vi "GV_Constructor.vi"(4 "Graph-ref":refnum<vi>, 5 "menu reference":refnum<k9>, 6 "StartupTagList":string[](array[string]), 7 "Pane":refnum<vi>, 8 "error in (no error)":errorcluster, 9 "Gserver-Queue":refnum<queue>, 10 "GviewName":string, 11 "Gviewer in":refnum<class "Gviewer.lvclass">) -> (0 "error out":errorcluster, 3 "Gviewer out":refnum<class "Gviewer.lvclass">)   [LabVIEW 2020, in "Sgraph_lib_V1.lvlib" / "Gviewer.lvclass"]
doc: "Constructor of the Sgraph Viewer : Set all default values, connect to Vserver, Setup default start conditions"
uses:
  Gviewer.lvclass
  Gserver/controls/Typedef_Gviewer-Query.ctl
  Gserver/controls/Typedef_QueryType.ctl
  Gviewer.lvclass/Gviewer.ctl
  <vilib>/Utility/miscctls.llb/LVPointTypeDef.ctl
  controls/ToolBarAppearance.ctl
  <vilib>/Utility/miscctls.llb/LVPositionTypeDef.ctl
  controls/Typedef_Gserver-Replies.ctl
  controls/Typedef_ServerActions.ctl
  FAMM/controls/Typedef_Gviewer_TagsUnits.ctl
  Common/controls/typedef_com_TagProp.ctl
  controls/TD_Lscale.ctl
  controls/TD_Rscale.ctl
  controls/Typedef_Live.ctl
  controls/MinMax.ctl
  controls/Typedef_ZoomEvent.ctl
  controls/Typedef_SelProperties.ctl
  controls/Typedef_LineType.ctl
  Gserver/Gserver.lvclass
  Builds/Sgraph_lib_V1.lvlib
  FAMM/FAMM.lvclass
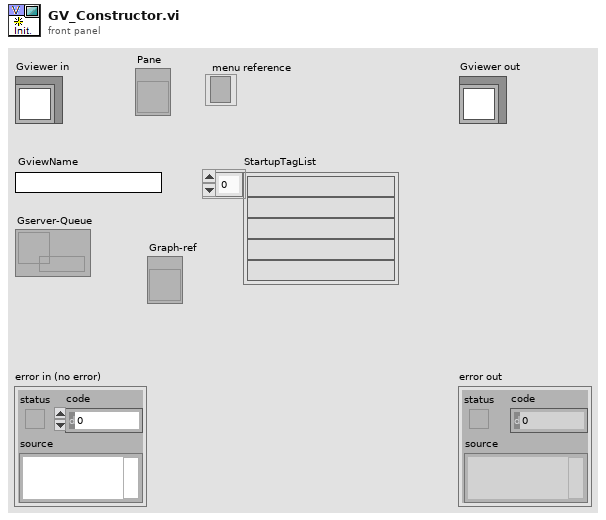
[diagram p1: front panel]
types:
  T1 = typedef "Sgraph_lib_V1.lvlib/Gviewer.lvclass/ToolBarAppearance.ctl" = enum16{"Bare", "Native", "Gradient"}
  T2 = typedef "LVPointTypeDef.ctl" = cluster{"Horizontal":i16, "Vertical":i16}
  T3 = typedef "LVPositionTypeDef.ctl" = cluster{"Left":i32, "Top":i32}
  T4 = typedef "Typedef_Gserver-Replies.ctl" = cluster{"ServerActions":T5, "data":variant, "Source":string, "Time Stamp":timestamp}
  T5 = typedef "Sgraph_lib_V1.lvlib/Gviewer.lvclass/Typedef_ServerActions.ctl" = enum16{"GraphUpdate", "SendAllTags", "SendIniPath", "SetGeneralOptions", "EditTagsOpen", "EditTagsPresetSave", "EditTagsPresetLoad", "EditTagsClose", "NewTagSelection", "AutoScale", "DBeditStatus", "DBsaveConfirm", "ExitGraph"}
  T6 = typedef "Sgraph_lib_V1.lvlib/Gserver.lvclass/Typedef_QueryType.ctl" = enum16{"Subscribe", "DataRequest", "RequestAllTags", "RequestIniPath", "FAMMstarted", "SetClientOptions", "GviewerUpdate", "OpenNewGraph", "CloseClient", "CloseAllClients", "Close Gserver", "OpenMemoryMap", "MeMapDataRequest", "MeMapDataResponse", "OpenDBeditor", "CheckDBeditorRunning", "StoppedDBeditor", "SaveDB_TAGpropRecord", "ConfirmDB_TAGpropSave"}
  T7 = typedef "Sgraph_lib_V1.lvlib/Gserver.lvclass/Typedef_Gviewer-Query.ctl" = cluster{"Query_type":T6, "data":variant, "Source":string, "Time Stamp":timestamp}
  T8 = enum32{"Invalid", "Standard", "Closed", "Hidden", "Minimized", "Maximized"}
  T9 = typedef "Sgraph_lib_V1.lvlib/FAMM.lvclass/Typedef_Gviewer_TagsUnits.ctl" = cluster{"PAQ_TAGs":string[], "WAQ_TAGs":string[], "EAQ_TAGs":string[], "PAQtagProps":T10[], "WAQtagProps":T10[], "EAQtagProps":T10[]}
  T10 = typedef "Sgraph_lib_V1.lvlib/typedef_com_TagProp.ctl" = cluster{"Description":string, "EngUnits":string, "RangeH":dbl, "RangeL":dbl, "Resolution":i32, "Obsolete":bool, "ChangeDate":timestamp, "ChangeSource":string, "ChangeReason":string, "TagFunc":u32}
  T11 = typedef "Sgraph_lib_V1.lvlib/Gviewer.lvclass/TD_Rscale.ctl" = enum16{"none", "one", "all"}
  T12 = typedef "Sgraph_lib_V1.lvlib/Gviewer.lvclass/TD_Lscale.ctl" = enum16{"none", "one", "many"}
  T13 = typedef "Sgraph_lib_V1.lvlib/Gviewer.lvclass/Typedef_Live.ctl" = enum16{"Live View", "Freeze"}
  T14 = typedef "Sgraph_lib_V1.lvlib/Gviewer.lvclass/MinMax.ctl" = enum16{"On", "Off", "Focus"}
  T15 = typedef "MenuStructure.ctl" = cluster{"After_tag":string, "MenuItems":T16[]}[]
  T16 = typedef "MenuItem.ctl" = cluster{"name":string, "tag":string, "checked":bool, "enabled":bool}
  T17 = typedef "Sgraph_lib_V1.lvlib/Gviewer.lvclass/Typedef_ZoomEvent.ctl" = cluster{"Time-Start":timestamp, "Time-End":timestamp, "TimeSpan(sec)":dbl, "Live":T13, "SelProperties":T18[], "Time Stamp":timestamp}
  T18 = typedef "Sgraph_lib_V1.lvlib/Gviewer.lvclass/Typedef_SelProperties.ctl" = cluster{"Color":u32, "LineType":T19, "max":dbl, "min":dbl, "unit":string}
  T19 = typedef "Sgraph_lib_V1.lvlib/Gviewer.lvclass/Typedef_LineType.ctl" = enum16{"num_bare", "num_MinMax_Area", "num_MinMax_Lines", "num_MinMax_Forfor", "num_Max_Area", "num_Max_Line", "num_Max_Forfor", "num_Min_Area", "num_Min_Line", "num_Min_Fosfor", "Boolean_Line_01", "Boolean_Area_01", "Boolean_Fosfor_01", "Boolean_Line_TF", "Boolean_Area_TF", "Boolean_Fosfor_TF", "Boolean_OnOff_Line", "Boolean_OnOff_Area", "Boolean_OnOff_Fosfor", "Boolean_spare", "StringEvent_Line", "StringEvent_TimeLine"}
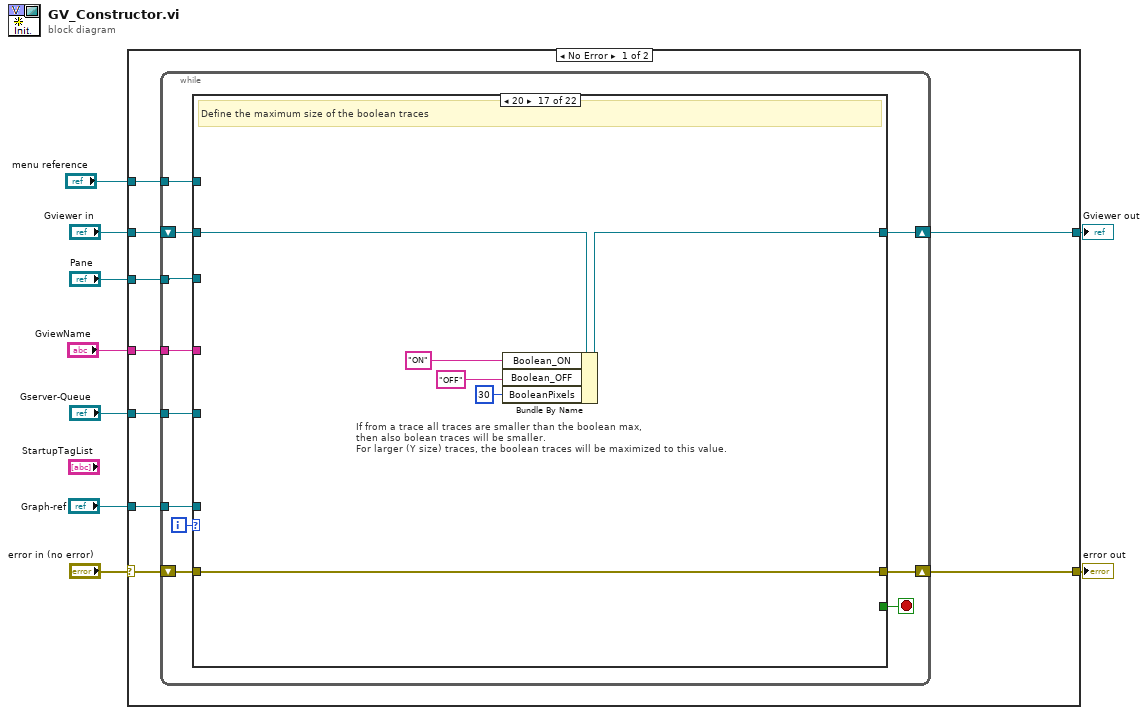
[diagram p0: block diagram]
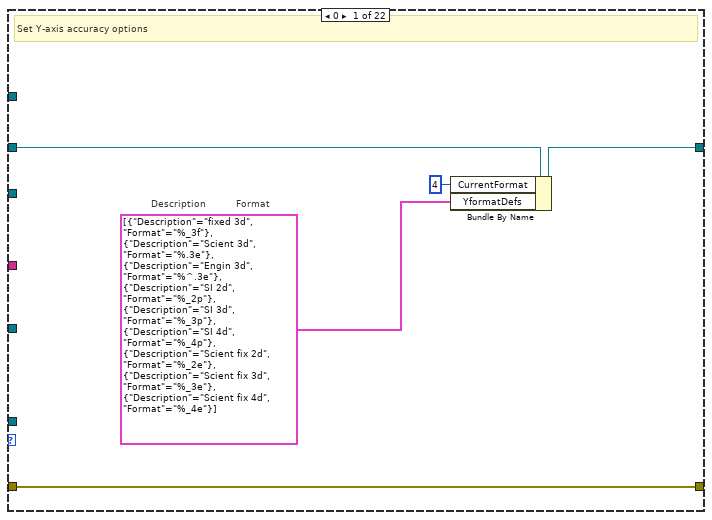
[diagram p2: hidden frame]
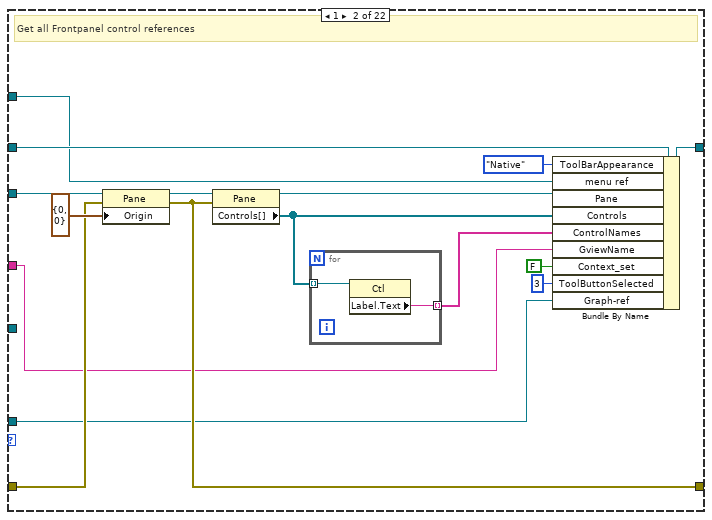
[diagram p3: hidden frame]
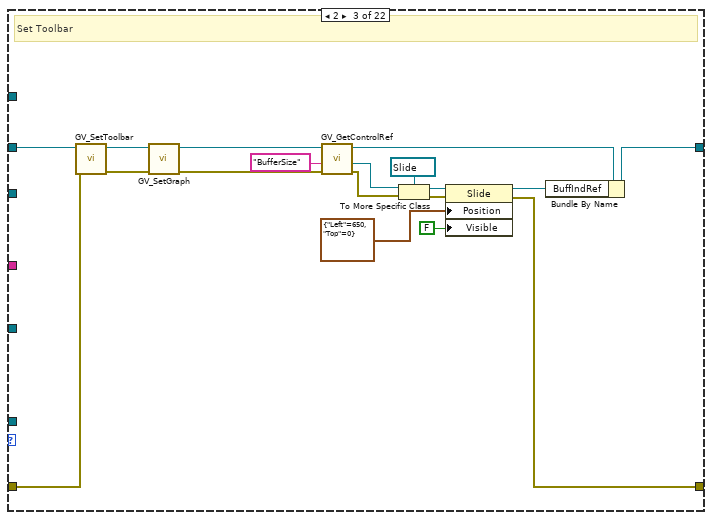
[diagram p4: hidden frame]
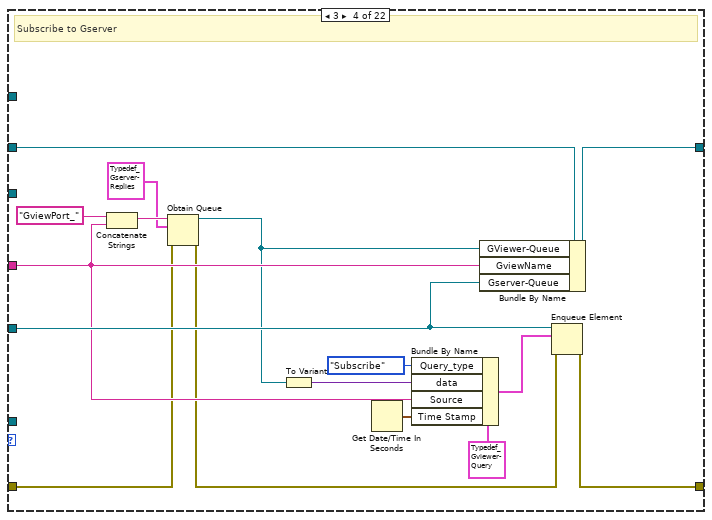
[diagram p5: hidden frame]
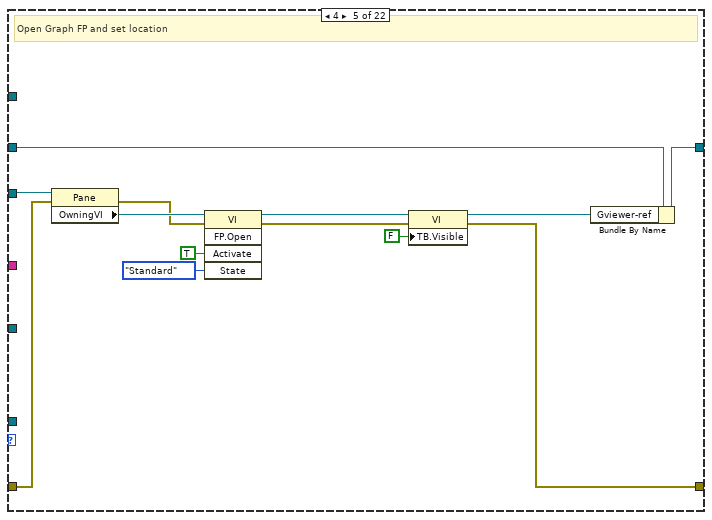
[diagram p6: hidden frame]
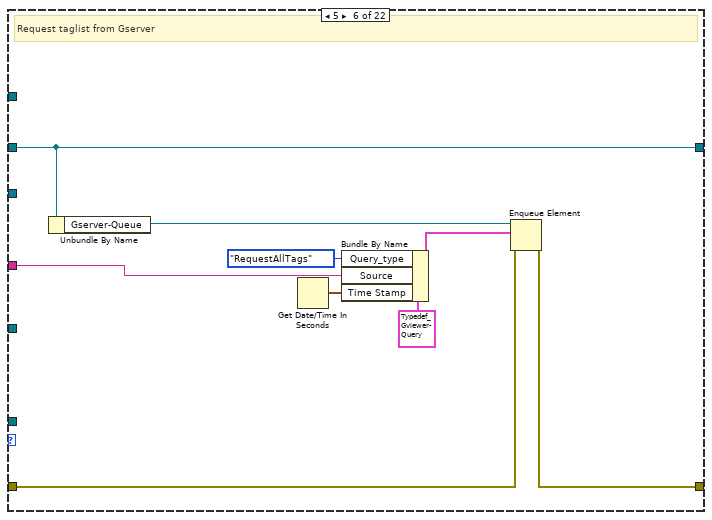
[diagram p7: hidden frame]
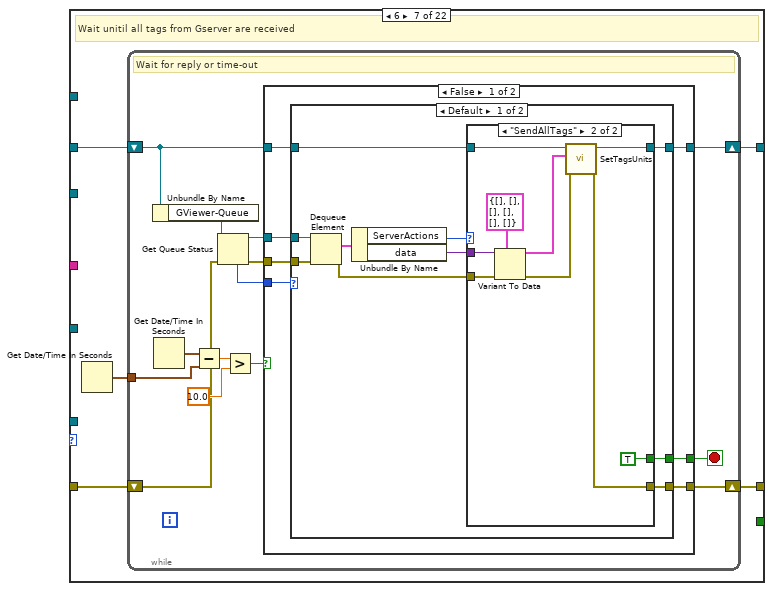
[diagram p8: hidden frame]
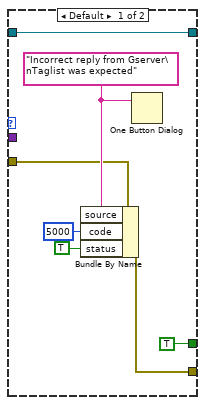
[diagram p9: hidden frame]
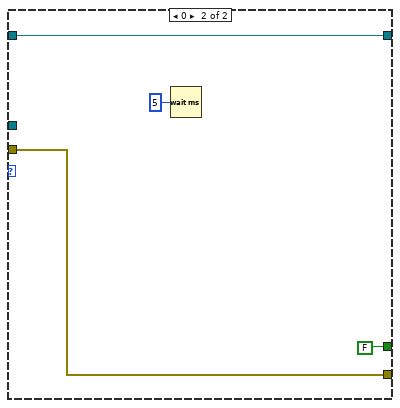
[diagram p10: hidden frame]
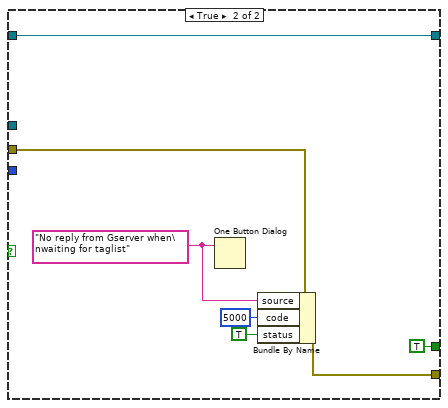
[diagram p11: hidden frame]
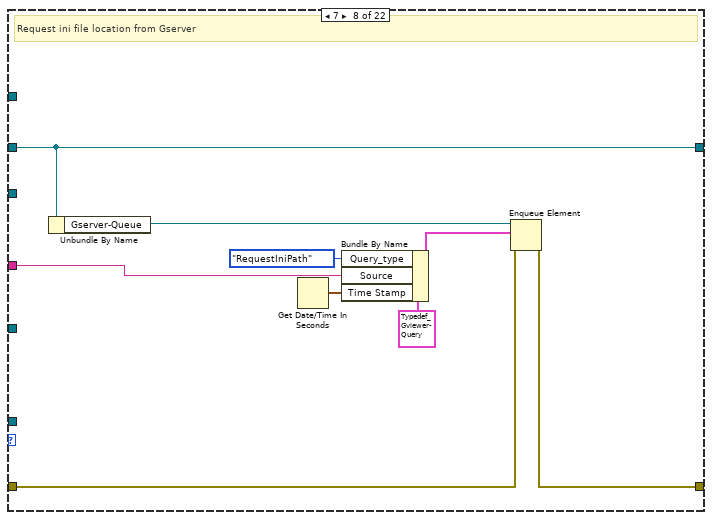
[diagram p12: hidden frame]
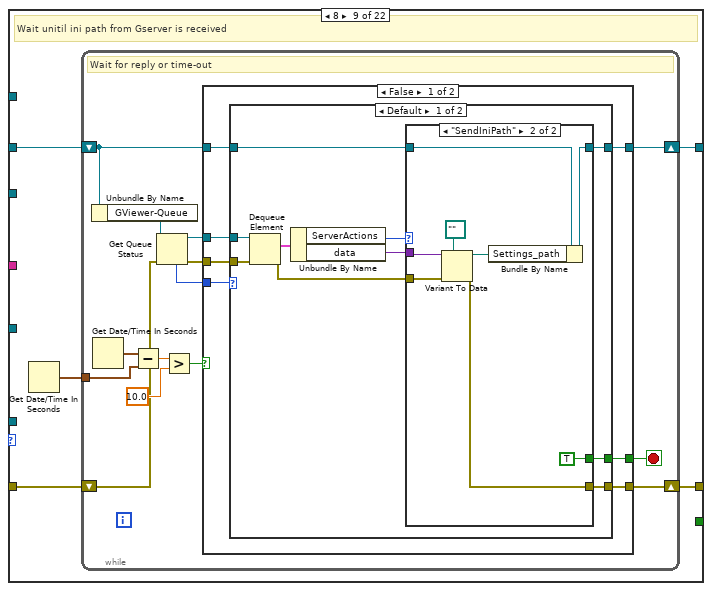
[diagram p13: hidden frame]
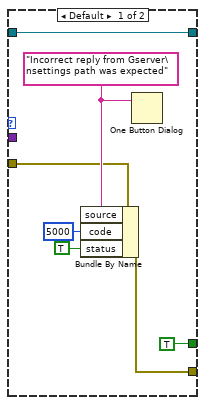
[diagram p14: hidden frame]
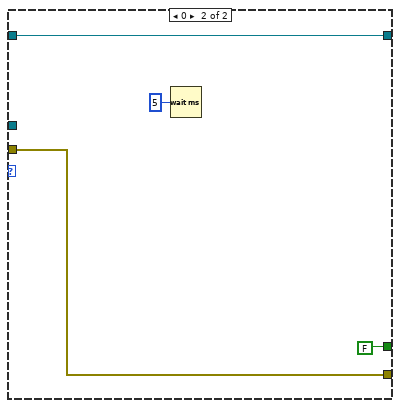
[diagram p15: hidden frame]
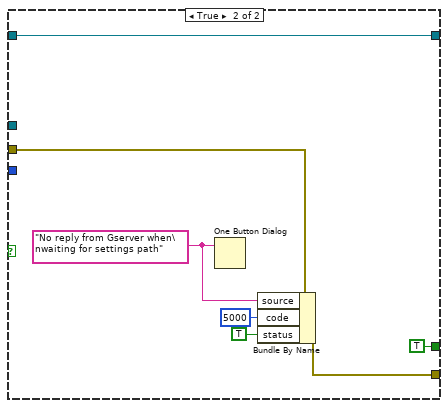
[diagram p16: hidden frame]
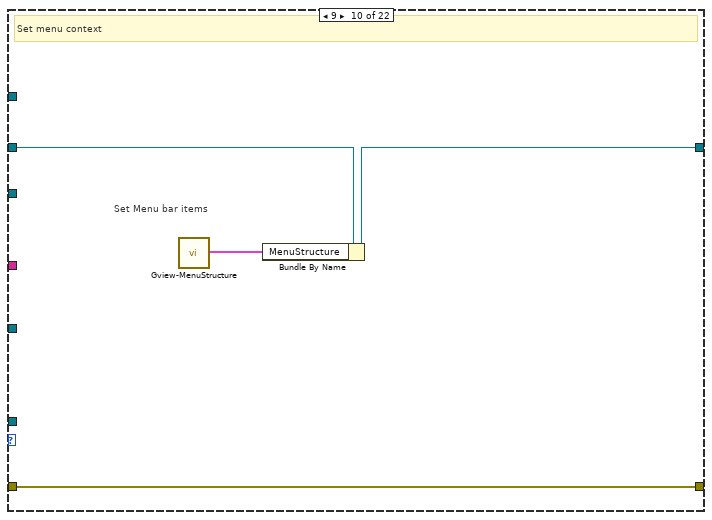
[diagram p17: hidden frame]
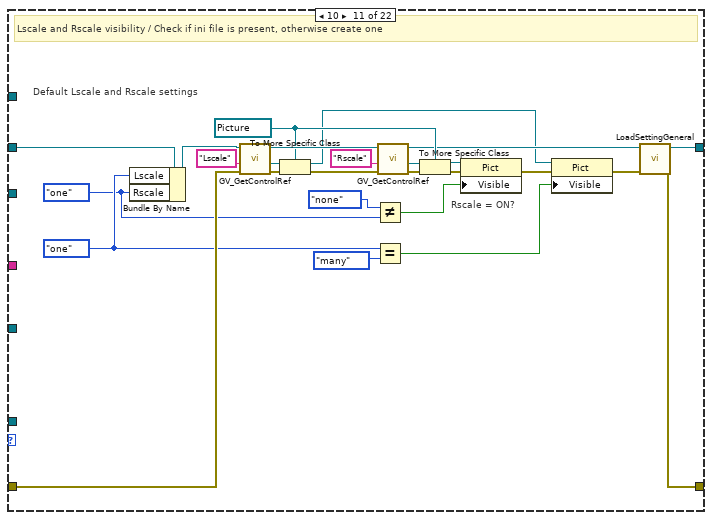
[diagram p18: hidden frame]
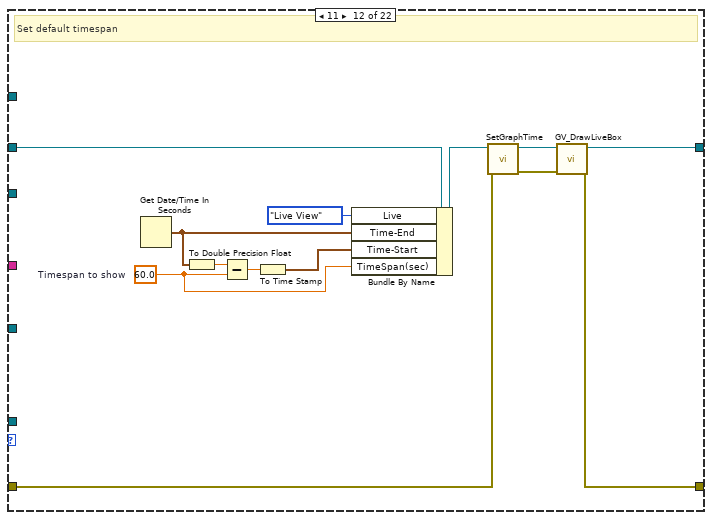
[diagram p19: hidden frame]
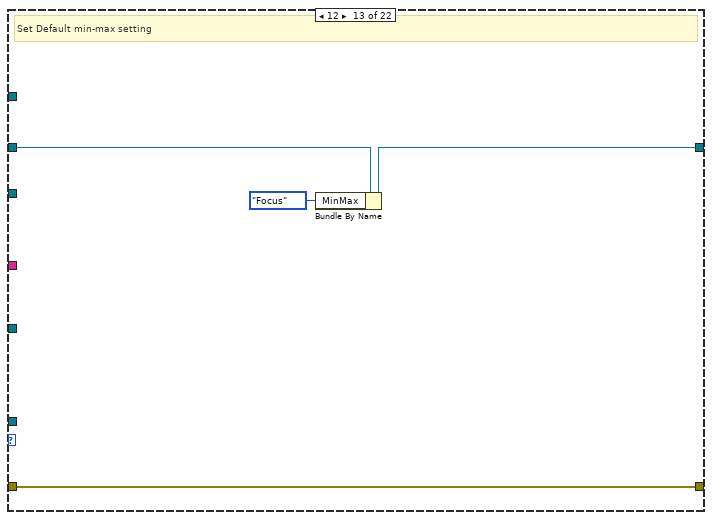
[diagram p20: hidden frame]
diagram:
  n1 = case shown="No Error" "error in (no error)" {
    selector: "error in (no error)" -> [w16 w347]
    tunnel: [w14 w347] -> w8
    tunnel: [w15 w346] -> w6
    tunnel: "Gviewer in" -> [w17 w346]
    tunnel: "Pane" -> [w18 _]
    tunnel: "GviewName" -> [w13 _]
    tunnel: "Gserver-Queue" -> [w12 _]
    tunnel: "menu reference" -> [w11 _]
    tunnel: "Graph-ref" -> [w10 _]
    frame No Error {
      n2 = while {
        tunnel: w18 -> [w25]
        shift-right: [w20] -> w15
        shift-left: w17 -> [w27]
        shift-right: [w28] -> w14
        shift-left: w16 -> [w19]
        tunnel: w13 -> [w24]
        tunnel: w12 -> [w23]
        tunnel: w11 -> [w22]
        tunnel: w10 -> [w21]
        i -> [w29]
        stop <- w26 stop-if-true
        n3 = case shown="20" w29 {
          tunnel: [w34 w46 w54 w83 w89 w103 w109 w175 w181 w243 w271 w274 w286 w291 w296 w299 w305 w310 w316 w334 w339 w344] -> w28
          tunnel: w27 -> [w32 w45 w70 w85 w92 w108 w112 w180 w184 w246 w270 w285 w289 w294 w297 w302 w308 w311 w322 w332 w342 w343]
          tunnel: [w33 w44 w56 w86 w93 w108 w111 w180 w183 w244 w272 w275 w288 w292 w298 w301 w307 w312 w314 w337 w341 w343] -> w20
          tunnel: [_ _ _ _ _ _ _ _ _ _ _ _ _ _ _ _ _ _ _ _ _ TRUE] -> w26
          tunnel: w25 -> [_ w50 _ _ w99 _ _ _ _ _ _ _ _ _ _ _ _ _ _ _ _ _]
          tunnel: w24 -> [_ w40 _ w77 _ w101 _ w173 _ _ _ _ _ _ _ _ _ _ _ _ _ _]
          tunnel: w23 -> [_ _ _ w84 _ _ _ _ _ _ _ _ _ _ _ _ _ _ _ _ _ _]
          tunnel: w22 -> [_ w39 _ _ _ _ _ _ _ _ _ _ _ _ _ _ _ _ _ _ _ _]
          tunnel: w21 -> [_ w35 _ _ _ _ _ _ _ _ _ _ _ _ _ _ _ _ _ _ _ _]
          tunnel: w19 -> [w34 w48 w69 w74 w98 w102 w110 w174 w182 w243 w258 w278 w286 w290 w295 w300 w305 w309 w318 w335 w340 w344]
          frame 0 {
            # "Description          Format"
            # "Set Y-axis accuracy options"
            n4 = Bundle By Name(cluster=w32, "CurrentFormat"=4, "YformatDefs"=cluster{"Description":string, "Format":string}[] [{"Description"="fixed 3d", "Format"="%_3f"}, {"Description"="Scient 3d", "Format"="%.3e"}, {"Description"="Engin 3d", "Format"="%^.3e"}, {"Description"="SI 2d", "Format"="%_2p"}, {"Description"="SI 3d", "Format"="%_3p"}, {"Description"="SI 4d", "Format"="%_4p"}, {"Description"="Scient fix 2d", "Format"="%_2e"}, {"Description"="Scient fix 3d", "Format"="%_3e"}, {"Description"="Scient fix 4d", "Format"="%_4e"}]) -> (w33:refnum<class "Gviewer.lvclass">)
          }
          frame 1 {
            # "Get all Frontpanel control references"
            n5 = property class="Pane"(reference=w50, error in=w48, "Origin"=T2 {"Horizontal"=0, "Vertical"=0}) -> (reference out=w47:refnum<vi>, error out=w46:errorcluster)
            n6 = property class="Pane"(reference=w47, error in=w46) -> (reference out=w41:refnum<vi>, "Controls[]"=w43:refnum<vi>[])  [unwired: 1 out]
            n7 = for {
              tunnel: w43 -> [w52] mode=indexing
              tunnel: [w51] -> w42 mode=indexing
              n8 = property class="Ctl"(reference=w52) -> ("Label.Text"=w51:string)  [unwired: 1 in, 2 out]
            }
            n9 = Bundle By Name(cluster=w45, "ToolBarAppearance"=ToolBarAppearance."Native", "menu ref"=w39, "Pane"=w41, "Controls"=w43, "ControlNames"=w42, "GviewName"=w40, "Context_set"=FALSE, "ToolButtonSelected"=3, "Graph-ref"=w35) -> (w44:refnum<class "Gviewer.lvclass">)
          }
          frame 2 {
            # "Set Toolbar"
            n10 = call "GV_SetToolbar.vi"("error in (no error)"=w69, "Gviewer in"=w70) -> ("error out"=w67:errorcluster, "Gviewer out"=w68:refnum<class "Gviewer.lvclass">)  [unwired: 8 in]
            n11 = call "GV_SetGraph.vi"("error in (no error)"=w67, "Gviewer in"=w68) -> ("error out"=w64:errorcluster, "Gviewer out"=w65:refnum<class "Gviewer.lvclass">)  [unwired: 8 in]
            n12 = call "GV_GetControlRef.vi"("error in (no error)"=w64, "CNT name"="BufferSize", "Gviewer in"=w65) -> ("error out"=w62:errorcluster, "Reference"=w63:refnum<vi>, "Gviewer out"=w57:refnum<class "Gviewer.lvclass">)  [unwired: 6 in]
            n13 = To More Specific Class(target class=refnum<vi> refnum ("BufferSize"), reference=w63, error in=w62) -> (specific class reference=w60:refnum<vi>, error out=w59:errorcluster)
            n14 = property class="Slide"(reference=w60, error in=w59, "Position"=T3 {"Left"=650, "Top"=0}, "Visible"=FALSE) -> (reference out=w58:refnum<vi>, error out=w54:errorcluster)
            n15 = Bundle By Name(cluster=w57, "BuffIndRef"=w58) -> (w56:refnum<class "Gviewer.lvclass">)
          }
          frame 3 {
            # "Subscribe to Gserver"
            n16 = Concatenate Strings("GviewPort_", w77) -> (w76:string)
            n17 = Obtain Queue(name (unnamed)=w76, element data type=T4 {"ServerActions"=enum."GraphUpdate", "data"=variant, "Source"="", "Time Stamp"=timestamp(0 s since 1904-01-01)} ("Query"), error in (no error)=w74) -> (queue out=w71:refnum<queue>, error out=w75:errorcluster)  [unwired: 2 in, 1 out]
            n18 = To Variant(anything=w71) -> (Variant=w72:variant)
            n19 = Get Date/Time In Seconds() -> (seconds since 1Jan1904=w79:timestamp)
            n20 = Bundle By Name(cluster=T7 {"Query_type"=enum."Subscribe", "data"=variant, "Source"="", "Time Stamp"=timestamp(0 s since 1904-01-01)} ("element"), "Query_type"=Typedef_QueryType."Subscribe", "data"=w72, "Source"=w77, "Time Stamp"=w79) -> (w81:T7)
            n21 = Bundle By Name(cluster=w85, "GViewer-Queue"=w71, "GviewName"=w77, "Gserver-Queue"=w84) -> (w86:refnum<class "Gviewer.lvclass">)
            n22 = Enqueue Element(queue=w84, element=w81, error in (no error)=w75) -> (error out=w83:errorcluster)  [unwired: 1 in, 2 out]
          }
          frame 4 {
            # "Open Graph FP and set location"
            n23 = property class="Pane"(reference=w99, error in=w98) -> (error out=w96:errorcluster, "OwningVI"=w97:refnum<vi>)  [unwired: 1 out]
            n24 = invoke class="VI" method="FP.Open"(reference=w97, error in=w96, "Activate"=TRUE ("Activate?"), "State"=T8."Standard") -> (reference out=w88:refnum<vi>, error out=w87:errorcluster)  [unwired: 1 in, 3 out]
            n25 = property class="VI"(reference=w88, error in=w87, "TB.Visible"=FALSE ("Tool Bar:Visible")) -> (reference out=w90:refnum<vi>, error out=w89:errorcluster)
            n26 = Bundle By Name(cluster=w92, "Gviewer-ref"=w90) -> (w93:refnum<class "Gviewer.lvclass">)
          }
          frame 5 {
            # "Request taglist from Gserver"
            n27 = Unbundle By Name(w108) -> ("Gserver-Queue"=w105:refnum<queue>)
            n28 = Get Date/Time In Seconds() -> (seconds since 1Jan1904=w100:timestamp)
            n29 = Bundle By Name(cluster=T7 {"Query_type"=enum."Subscribe", "data"=variant, "Source"="", "Time Stamp"=timestamp(0 s since 1904-01-01)} ("element"), "Query_type"=Typedef_QueryType."RequestAllTags", "Source"=w101, "Time Stamp"=w100) -> (w104:T7)
            n30 = Enqueue Element(queue=w105, element=w104, error in (no error)=w102) -> (error out=w103:errorcluster)  [unwired: 1 in, 2 out]
          }
          frame 6 {
            # "Wait unitil all tags from Gserver are received"
            n31 = Get Date/Time In Seconds() -> (seconds since 1Jan1904=w113:timestamp)
            n32 = while {
              tunnel: w113 -> [w126]
              shift-right: [w122] -> w111
              shift-left: w112 -> [w119]
              shift-right: [w121] -> w109
              shift-left: w110 -> [w115]
              stop <- w120 stop-if-true
              # "Wait for reply or time-out"
              n33 = Unbundle By Name(w119) -> ("GViewer-Queue"=w118:refnum<queue>)
              n34 = Get Date/Time In Seconds() -> (seconds since 1Jan1904=w127:timestamp)
              n35 = Subtract(x=w127, y=w126) -> (x-y=w125:dbl)
              n36 = Get Queue Status(queue=w118, error in (no error)=w115) -> (queue out=w117:refnum<queue>, error out=w114:errorcluster, # elements in queue=w116:i32)  [unwired: 1 in, 5 out]
              n37 = Greater?(x=w125, y=10.0) -> (0:w123:bool)
              n38 = case shown="False" w123 {
                tunnel: w119 -> [w133 w171]
                tunnel: [w132 w171] -> w122
                tunnel: [w131 w167] -> w121
                tunnel: [w128 TRUE] -> w120
                tunnel: w117 -> [w130 _]
                tunnel: w116 -> [w134 _]
                tunnel: w114 -> [w129 w166]
                frame False {
                  n39 = case shown="Default" w134 {
                    tunnel: w133 -> [w140 w164]
                    tunnel: [w139 w164] -> w132
                    tunnel: [w138 w162] -> w131
                    tunnel: w130 -> [w143 _]
                    tunnel: w129 -> [w142 w162]
                    tunnel: [w136 FALSE] -> w128
                    frame Default {
                      n40 = Dequeue Element(queue=w143, error in (no error)=w142) -> (element=w144:T4, error out=w137:errorcluster)  [unwired: 1 in, 2 out]
                      n41 = Unbundle By Name(w144) -> ("ServerActions"=w141:T5, "data"=w135:variant)
                      n42 = case shown="\"SendAllTags\"" w141 {
                        tunnel: w140 -> [w151 w156]
                        tunnel: [w151 w155] -> w139
                        tunnel: [w146 w152] -> w138
                        tunnel: w137 -> [w145 w158]
                        tunnel: [TRUE TRUE] -> w136
                        tunnel: w135 -> [_ w159]
                        frame Default {
                          w147 = "Incorrect reply from Gserver\nTaglist was expected" ("message")
                          n43 = Bundle By Name(cluster=w145, "source"=w147, "code"=5000, "status"=TRUE) -> (w146:errorcluster)
                          n44 = One Button Dialog(message=w147) -> ()  [unwired: 1 in, 1 out]
                        }
                        frame "SendAllTags" {
                          n45 = Variant To Data(error in=w158, type=T9 {"PAQ_TAGs"=[], "WAQ_TAGs"=[], "EAQ_TAGs"=[], "PAQtagProps"=[], "WAQtagProps"=[], "EAQtagProps"=[]} ("Tags_Units"), Variant=w159) -> (data=w154:T9, error out=w153:errorcluster)
                          n46 = call "SetTagsUnits.vi"("error in (no error)"=w153, "Tags_Units"=w154, "Gviewer in"=w156) -> ("error out"=w152:errorcluster, "Gviewer out"=w155:refnum<class "Gviewer.lvclass">)  [unwired: 7 in]
                        }
                      }
                    }
                    frame 0 {
                      n47 = Wait (ms)(milliseconds to wait=u32 5) -> ()  [unwired: 1 out]
                    }
                  }
                }
                frame True {
                  w165 = "No reply from Gserver when\nwaiting for taglist" ("message")
                  n48 = One Button Dialog(message=w165) -> ()  [unwired: 1 in, 1 out]
                  n49 = Bundle By Name(cluster=w166, "source"=w165, "code"=5000, "status"=TRUE) -> (w167:errorcluster)
                }
              }
            }
          }
          frame 7 {
            # "Request ini file location from Gserver"
            n50 = Unbundle By Name(w180) -> ("Gserver-Queue"=w177:refnum<queue>)
            n51 = Get Date/Time In Seconds() -> (seconds since 1Jan1904=w172:timestamp)
            n52 = Bundle By Name(cluster=T7 {"Query_type"=enum."Subscribe", "data"=variant, "Source"="", "Time Stamp"=timestamp(0 s since 1904-01-01)} ("element"), "Query_type"=Typedef_QueryType."RequestIniPath", "Source"=w173, "Time Stamp"=w172) -> (w176:T7)
            n53 = Enqueue Element(queue=w177, element=w176, error in (no error)=w174) -> (error out=w175:errorcluster)  [unwired: 1 in, 2 out]
          }
          frame 8 {
            # "Wait unitil ini path from Gserver is received"
            n54 = Get Date/Time In Seconds() -> (seconds since 1Jan1904=w185:timestamp)
            n55 = while {
              tunnel: w185 -> [w198]
              shift-right: [w194] -> w183
              shift-left: w184 -> [w191]
              shift-right: [w193] -> w181
              shift-left: w182 -> [w187]
              stop <- w192 stop-if-true
              # "Wait for reply or time-out"
              n56 = Unbundle By Name(w191) -> ("GViewer-Queue"=w190:refnum<queue>)
              n57 = Get Date/Time In Seconds() -> (seconds since 1Jan1904=w199:timestamp)
              n58 = Subtract(x=w199, y=w198) -> (x-y=w197:dbl)
              n59 = Get Queue Status(queue=w190, error in (no error)=w187) -> (queue out=w189:refnum<queue>, error out=w186:errorcluster, # elements in queue=w188:i32)  [unwired: 1 in, 5 out]
              n60 = Greater?(x=w197, y=10.0) -> (0:w195:bool)
              n61 = case shown="False" w195 {
                tunnel: w191 -> [w205 w242]
                tunnel: [w204 w242] -> w194
                tunnel: [w203 w238] -> w193
                tunnel: [w200 TRUE] -> w192
                tunnel: w189 -> [w202 _]
                tunnel: w188 -> [w206 _]
                tunnel: w186 -> [w201 w237]
                frame False {
                  n62 = case shown="Default" w206 {
                    tunnel: w205 -> [w212 w235]
                    tunnel: [w211 w235] -> w204
                    tunnel: [w210 w233] -> w203
                    tunnel: w202 -> [w215 _]
                    tunnel: w201 -> [w214 w233]
                    tunnel: [w208 FALSE] -> w200
                    frame Default {
                      n63 = Dequeue Element(queue=w215, error in (no error)=w214) -> (element=w216:T4, error out=w209:errorcluster)  [unwired: 1 in, 2 out]
                      n64 = Unbundle By Name(w216) -> ("ServerActions"=w213:T5, "data"=w207:variant)
                      n65 = case shown="\"SendIniPath\"" w213 {
                        tunnel: w212 -> [w223 w229]
                        tunnel: [w223 w228] -> w211
                        tunnel: [w218 w226] -> w210
                        tunnel: w209 -> [w217 w225]
                        tunnel: [TRUE TRUE] -> w208
                        tunnel: w207 -> [_ w227]
                        frame Default {
                          w219 = "Incorrect reply from Gserver\nsettings path was expected" ("message")
                          n66 = Bundle By Name(cluster=w217, "source"=w219, "code"=5000, "status"=TRUE) -> (w218:errorcluster)
                          n67 = One Button Dialog(message=w219) -> ()  [unwired: 1 in, 1 out]
                        }
                        frame "SendIniPath" {
                          n68 = Variant To Data(error in=w225, type=path "" ("Path"), Variant=w227) -> (data=w230:path, error out=w226:errorcluster)
                          n69 = Bundle By Name(cluster=w229, "Settings_path"=w230) -> (w228:refnum<class "Gviewer.lvclass">)
                        }
                      }
                    }
                    frame 0 {
                      n70 = Wait (ms)(milliseconds to wait=u32 5) -> ()  [unwired: 1 out]
                    }
                  }
                }
                frame True {
                  w236 = "No reply from Gserver when\nwaiting for settings path" ("message")
                  n71 = One Button Dialog(message=w236) -> ()  [unwired: 1 in, 1 out]
                  n72 = Bundle By Name(cluster=w237, "source"=w236, "code"=5000, "status"=TRUE) -> (w238:errorcluster)
                }
              }
            }
          }
          frame 9 {
            # "Set Menu bar items"
            # "Set menu context"
            n73 = call "Gview-MenuStructure.vi"() -> ("MenuStructure"=w245:T15)  [unwired: 2 in]
            n74 = Bundle By Name(cluster=w246, "MenuStructure"=w245) -> (w244:refnum<class "Gviewer.lvclass">)
          }
          frame 10 {
            w261 = refnum<vi> refnum ("2D Picture")
            w249 = TD_Rscale."one" ("Rscale")
            w252 = TD_Lscale."one" ("Lscale")
            # "Rscale = ON?"
            # "Default Lscale and Rscale settings"
            # "Lscale and Rscale visibility / Check if ini file is present, otherwise create one"
            n75 = Bundle By Name(cluster=w270, "Lscale"=w252, "Rscale"=w249) -> (w260:refnum<class "Gviewer.lvclass">)
            n76 = call "GV_GetControlRef.vi"("error in (no error)"=w258, "CNT name"="Lscale", "Gviewer in"=w260) -> ("error out"=w265:errorcluster, "Reference"=w266:refnum<vi>, "Gviewer out"=w269:refnum<class "Gviewer.lvclass">)  [unwired: 6 in]
            n77 = To More Specific Class(target class=w261, reference=w266, error in=w265) -> (specific class reference=w253:refnum<vi>, error out=w263:errorcluster)
            n78 = Not Equal?(x=TD_Rscale."none" ("Rscale"), y=w249) -> (x != y?=w248:bool)
            n79 = Equal?(x=w252, y=TD_Lscale."many" ("Lscale")) -> (x = y?=w250:bool)
            n80 = call "GV_GetControlRef.vi"("error in (no error)"=w263, "CNT name"="Rscale", "Gviewer in"=w269) -> ("error out"=w262:errorcluster, "Reference"=w264:refnum<vi>, "Gviewer out"=w259:refnum<class "Gviewer.lvclass">)  [unwired: 6 in]
            n81 = To More Specific Class(target class=w261, reference=w264, error in=w262) -> (specific class reference=w254:refnum<vi>, error out=w256:errorcluster)
            n82 = property class="Pict"(reference=w254, error in=w256, "Visible"=w248) -> (error out=w257:errorcluster)  [unwired: 1 out]
            n83 = property class="Pict"(reference=w253, error in=w257, "Visible"=w250) -> (error out=w255:errorcluster)  [unwired: 1 out]
            n84 = call "LoadSettingGeneral.vi"("error in (no error)"=w255, "Gviewer in"=w259) -> ("error out"=w271:errorcluster, "Gviewer out"=w272:refnum<class "Gviewer.lvclass">)  [unwired: 7 in, 1 out]
          }
          frame 11 {
            w280 = 60.0  # Timespan to show
            # "Set default timespan"
            n85 = Get Date/Time In Seconds() -> (seconds since 1Jan1904=w284:timestamp)
            n86 = To Double Precision Float(number=w284) -> (double precision float=w283:dbl)
            n87 = Subtract(x=w283, y=w280) -> (x-y=w282:dbl)
            n88 = To Time Stamp(1:w282) -> (0:w281:timestamp)
            n89 = Bundle By Name(cluster=w285, "Live"=Typedef_Live."Live View", "Time-End"=w284, "Time-Start"=w281, "TimeSpan(sec)"=w280) -> (w279:refnum<class "Gviewer.lvclass">)
            n90 = call "SetGraphTime.vi"("error in (no error)"=w278, "Gviewer in"=w279) -> ("error out"=w276:errorcluster, "Gviewer out"=w277:refnum<class "Gviewer.lvclass">)  [unwired: 8 in]
            n91 = call "GV_DrawLiveBox.vi"("error in (no error)"=w276, "Gviewer in"=w277) -> ("error out"=w274:errorcluster, "Gviewer out"=w275:refnum<class "Gviewer.lvclass">)  [unwired: 8 in]
          }
          frame 12 {
            # "Set Default min-max setting"
            n92 = Bundle By Name(cluster=w289, "MinMax"=MinMax."Focus") -> (w288:refnum<class "Gviewer.lvclass">)
          }
          frame 13 {
            # "Get Default TAG settings for this graph"
            n93 = call "Tag_settings_load.vi"("error in (no error)"=w290, "PresetName"="default" ("SettingsName"), "Gviewer in"=w294) -> ("error out"=w291:errorcluster, "Gviewer out"=w292:refnum<class "Gviewer.lvclass">)  [unwired: 7 in]
          }
          frame 14 {
            # "Set menu bar context"
            n94 = call "SetMenuBar.vi"("error in (no error)"=w295, "Gviewer in"=w297) -> ("error out"=w296:errorcluster, "Gviewer out"=w298:refnum<class "Gviewer.lvclass">)  [unwired: 8 in]
          }
          frame 15 {
            # "Set Graph TAG Properties"
            n95 = call "SetClassProperties.vi"("error in (no error)"=w300, "Gviewer in"=w302) -> ("error out"=w299:errorcluster, "Gviewer out"=w301:refnum<class "Gviewer.lvclass">)  [unwired: 8 in]
          }
          frame 20 {
            # "If from a trace all traces are smaller than the boolean max,\nthen also bolean traces will be smaller.\nFor larger (Y size) traces, the boolean traces will be maximized to this value."
            # "Define the maximum size of the boolean traces"
            n96 = Bundle By Name(cluster=w308, "Boolean_ON"="ON", "Boolean_OFF"="OFF", "BooleanPixels"=u16 30) -> (w307:refnum<class "Gviewer.lvclass">)
          }
          frame 16 {
            # "Request first frame from Gserver"
            n97 = call "Request_Gserver_Update.vi"("error in (no error)"=w309, "Gviewer in"=w311) -> ("error out"=w310:errorcluster, "Gviewer out"=w312:refnum<class "Gviewer.lvclass">)  [unwired: 8 in]
          }
          frame 17 {
            # "Determine if Legend is visible at startup"
            n98 = call "GV_LegendOnOff.vi"("error in (no error)"=w318, "On?"=FALSE, "Gviewer in"=w322) -> ("error out"=w319:errorcluster, "Visible?"=w320:bool, "Gviewer out"=w321:refnum<class "Gviewer.lvclass">)  [unwired: 6 in]
            n99 = call "SetMenuTagChecked.vi"("error in (no error)"=w319, "Checked"=w320, "TAG"="Legend", "Gviewer in"=w321) -> ("error out"=w324:errorcluster, "Gviewer out"=w325:refnum<class "Gviewer.lvclass">)  [unwired: 6 in]
            n100 = call "SetMenuBar.vi"("error in (no error)"=w324, "Gviewer in"=w325) -> ("error out"=w316:errorcluster, "Gviewer out"=w315:refnum<class "Gviewer.lvclass">)  [unwired: 8 in]
            n101 = Bundle By Name(cluster=w315, "PlotSelected"=-1) -> (w314:refnum<class "Gviewer.lvclass">)
          }
          frame 18 {
            w333 = T17 {"Time-Start"=timestamp(0 s since 1904-01-01), "Time-End"=timestamp(0 s since 1904-01-01), "TimeSpan(sec)"=0.0, "Live"=enum."Live View", "SelProperties"=[], "Time Stamp"=timestamp(0 s since 1904-01-01)} ("ZoomEvent")
            # "Add first default setting to undo memory"
            n102 = Unbundle By Name(w332) -> ("Time-Start"=w331:timestamp, "Time-End"=w330:timestamp, "TimeSpan(sec)"=w329:dbl, "Live"=w327:T13, "SelProperties"=w328:T18[])
            n103 = Get Date/Time In Seconds() -> (seconds since 1Jan1904=w326:timestamp)
            n104 = Bundle By Name(cluster=w333, "Time-Start"=w331, "Time-End"=w330, "TimeSpan(sec)"=w329, "Live"=w327, "SelProperties"=w328, "Time Stamp"=w326) -> ()  [unwired: 1 out]
            n105 = call "GV_Undo_add.vi"("error in (no error)"=w335, "ZoomEvent"=w333, "Gviewer in"=w332) -> ("error out"=w334:errorcluster, "Gviewer out"=w336:refnum<class "Gviewer.lvclass">)  [unwired: 7 in]
            n106 = Bundle By Name(cluster=w336, "MaxUndoDepth"=20) -> (w337:refnum<class "Gviewer.lvclass">)
          }
          frame 19 {
            # "Set Graph size based on Lscale and Rscale settings"
            n107 = call "GV_SetGraph.vi"("error in (no error)"=w340, "Gviewer in"=w342) -> ("error out"=w339:errorcluster, "Gviewer out"=w341:refnum<class "Gviewer.lvclass">)  [unwired: 8 in]
          }
          frame Default {
            # "Last init frame"
          }
        }
      }
    }
    frame Error {
    }
  }
  "error out" <- w8
  "Gviewer out" <- w6
